vi "LS370_set_control_values.vi"(1 "System Monitor Variables (in)":T1) -> (0 "System Monitor Variables (out)":T1)   [LabVIEW 2019]
uses:
  Global/Global Variables/System Monitor Cluster.ctl
  Global/Global Variables/Data_Display_global.vi
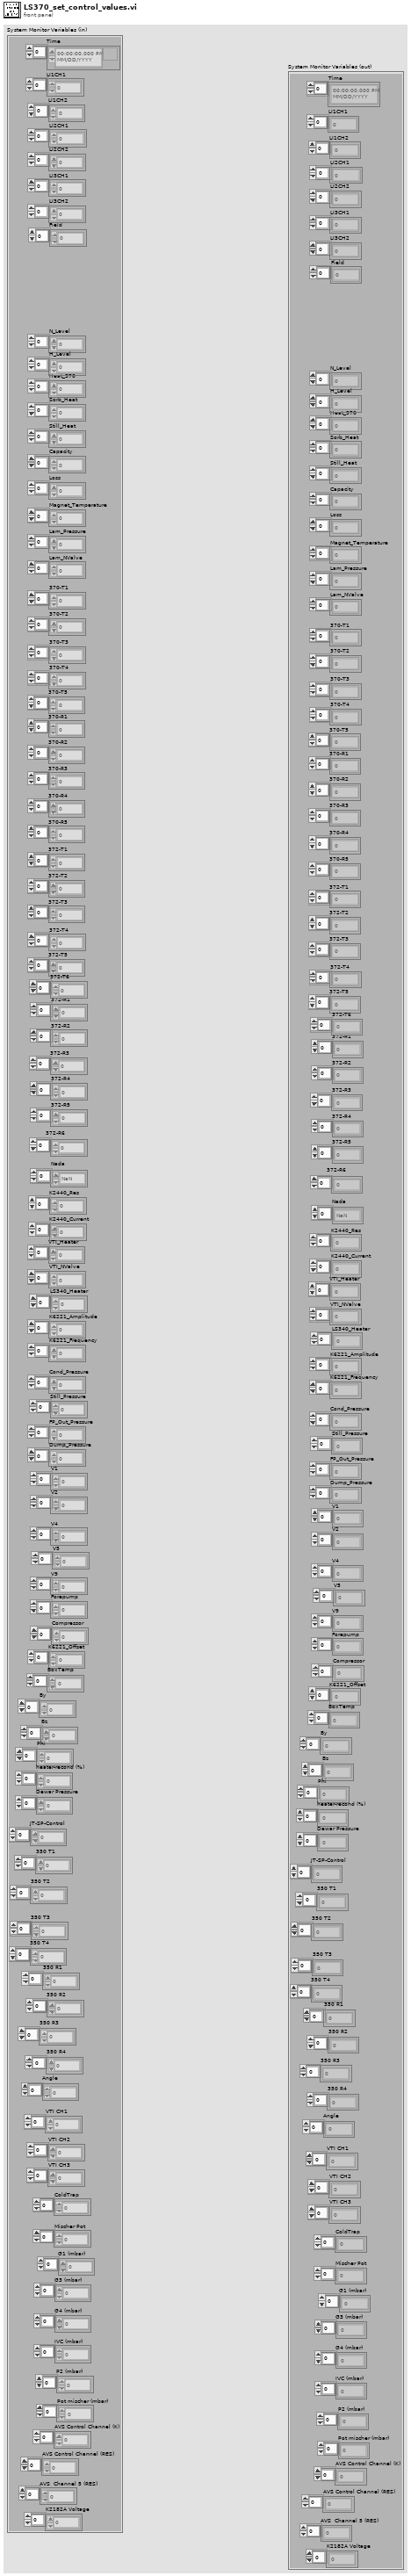
[diagram p1: front panel]
types:
  T1 = typedef "System Monitor Cluster.ctl" = cluster{"Time":timestamp[], "LI1CH1":dbl[], "LI1CH2":dbl[], "LI2CH1":dbl[], "LI2CH2":dbl[], "LI3CH1":dbl[], "LI3CH2":dbl[], "Field":dbl[], "N_Level":dbl[], "H_Level":dbl[], "Heat_370":dbl[], "Sorb_Heat":dbl[], "Still_Heat":dbl[], "Capacity":dbl[], "Loss":dbl[], "Magnet_Temperature":dbl[], "Lam_Pressure":dbl[], "Lam_NValve":dbl[], "370-T1":dbl[], "370-T2":dbl[], "370-T3":dbl[], "370-T4":dbl[], "370-T5":dbl[], "370-R1":dbl[], "370-R2":dbl[], "370-R3":dbl[], "370-R4":dbl[], "370-R5":dbl[], "372-T1":dbl[], "372-T2":dbl[], "372-T3":dbl[], "372-T4":dbl[], "372-T5":dbl[], "372-T6":dbl[], "372-R1":dbl[], "372-R2":dbl[], "372-R3":dbl[], "372-R4":dbl[], "372-R5":dbl[], "372-R6":dbl[], "Nada":dbl[], "K2440_Res":dbl[], "K2440_Current":dbl[], "VTI_Heater":dbl[], "VTI_NValve":dbl[], "LS340_Heater":dbl[], "K6221_Amplitude":dbl[], "K6221_Frequency":dbl[], "Cond_Pressure":dbl[], "Still_Pressure":dbl[], "FP_Out_Pressure":dbl[], "Dump_Pressure":dbl[], "V1":dbl[], "V2":dbl[], "V4":dbl[], "V5":dbl[], "V9":dbl[], "Forepump":dbl[], "Compressor":dbl[], "K6221_Offset":dbl[], "BoxTemp":dbl[], "By":dbl[], "Bz":dbl[], "Phi":dbl[], "heater-recond (%)":dbl[], "Dewar Pressure ":dbl[], "JT-SP-Control":dbl[], "350 T1":dbl[], "350 T2":dbl[], "350 T3":dbl[], "350 T4":dbl[], "350 R1":dbl[], "350 R2":dbl[], "350 R3":dbl[], "350 R4":dbl[], "Angle":dbl[], "VTI CH1":dbl[], "VTI CH2":dbl[], "VTI CH3":dbl[], "ColdTrap":dbl[], "Mischer Pot":dbl[], "G1 (mbar)":dbl[], "G3 (mbar) ":dbl[], "G4 (mbar)":dbl[], "IVC (mbar)":dbl[], "P2 (mbar) ":dbl[], "Pot mischer (mbar)":dbl[], "AVS Control Channel (K)":dbl[], "AVS Control Channel (RES)":dbl[], "AVS  Channel 5 (RES) ":dbl[], "K2182A Voltage":dbl[]}
  T2 = typedef "LS370_Status.ctl" = cluster{"Setpoint":dbl, "MC Heater Output":dbl, "Still Heater Output":dbl, "Sorb  Heater Output":dbl, "LS370 T1":dbl, "LS370 T2":dbl, "LS370 T3":dbl, "LS370 T4":dbl, "LS370 T5":dbl, "LS370 R1":dbl, "LS370 R2":dbl, "LS370 R3":dbl, "LS370 R4":dbl, "LS370 R5":dbl, "LS370 T6":dbl, "LS370 T7":dbl, "LS370 T8":dbl, "LS370 T9":dbl, "LS370 R6":dbl, "LS370 R7":dbl, "LS370 R8":dbl, "LS370 R9":dbl, "LS370 TC-T":dbl, "LS370 TC-R":dbl}
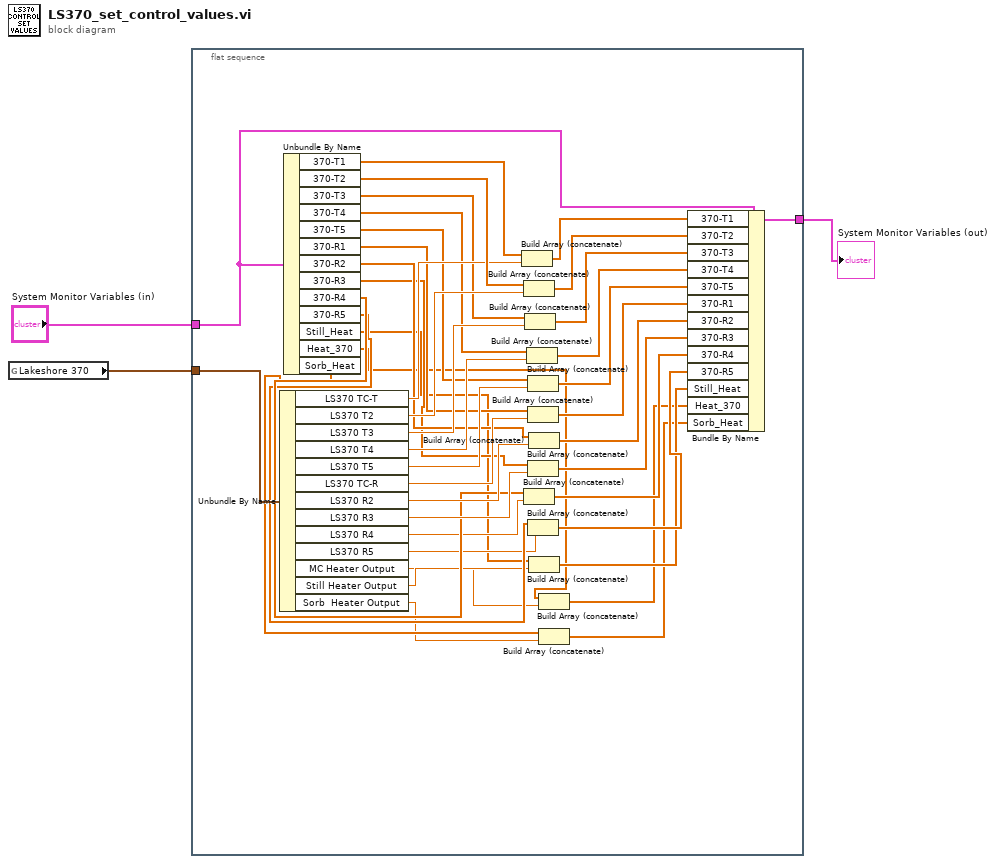
[diagram p0: block diagram]
diagram:
  n1 = global read "Data_Display_global.vi" "Lakeshore 370"() -> (w2:T2)
  n2 = flat-sequence {
    tunnel: "System Monitor Variables (in)" -> [w43]
    tunnel: w2 -> [w44]
    tunnel: [w45] -> w1
    frame #0 {
      n3 = Unbundle By Name(w44) -> ("LS370 TC-T"=w39:dbl, "LS370 T2"=w38:dbl, "LS370 T3"=w35:dbl, "LS370 T4"=w32:dbl, "LS370 T5"=w29:dbl, "LS370 TC-R"=w26:dbl, "LS370 R2"=w23:dbl, "LS370 R3"=w20:dbl, "LS370 R4"=w17:dbl, "LS370 R5"=w14:dbl, "MC Heater Output"=w8:dbl, "Still Heater Output"=w11:dbl, "Sorb  Heater Output"=w6:dbl)
      n4 = Unbundle By Name(w43) -> ("370-T1"=w42:dbl[], "370-T2"=w40:dbl[], "370-T3"=w36:dbl[], "370-T4"=w33:dbl[], "370-T5"=w30:dbl[], "370-R1"=w27:dbl[], "370-R2"=w24:dbl[], "370-R3"=w21:dbl[], "370-R4"=w18:dbl[], "370-R5"=w15:dbl[], "Still_Heat"=w12:dbl[], "Heat_370"=w9:dbl[], "Sorb_Heat"=w7:dbl[])
      n5 = Build Array (concatenate)(w42, w39) -> (w41:dbl[])
      n6 = Build Array (concatenate)(w40, w38) -> (w37:dbl[])
      n7 = Build Array (concatenate)(w18, w17) -> (w16:dbl[])
      n8 = Build Array (concatenate)(w36, w35) -> (w34:dbl[])
      n9 = Build Array (concatenate)(w33, w32) -> (w31:dbl[])
      n10 = Build Array (concatenate)(w30, w29) -> (w28:dbl[])
      n11 = Build Array (concatenate)(w27, w26) -> (w25:dbl[])
      n12 = Build Array (concatenate)(w21, w20) -> (w19:dbl[])
      n13 = Build Array (concatenate)(w15, w14) -> (w13:dbl[])
      n14 = Build Array (concatenate)(w24, w23) -> (w22:dbl[])
      n15 = Build Array (concatenate)(w12, w11) -> (w10:dbl[])
      n16 = Build Array (concatenate)(w9, w8) -> (w4:dbl[])
      n17 = Build Array (concatenate)(w7, w6) -> (w5:dbl[])
      n18 = Bundle By Name(cluster=w43, "370-T1"=w41, "370-T2"=w37, "370-T3"=w34, "370-T4"=w31, "370-T5"=w28, "370-R1"=w25, "370-R2"=w22, "370-R3"=w19, "370-R4"=w16, "370-R5"=w13, "Still_Heat"=w10, "Heat_370"=w4, "Sorb_Heat"=w5) -> (w45:T1)
    }
  }
  "System Monitor Variables (out)" <- w1
